vi "ERROR_DIALOGUE.vi"(0 "String":string) -> ()   [LabVIEW 2018]
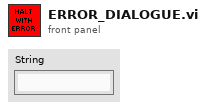
[diagram p1: front panel]
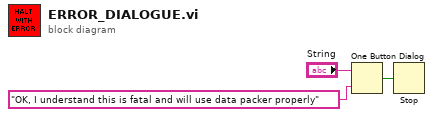
[diagram p0: block diagram]
diagram:
  n1 = One Button Dialog(message="String", button name ("OK")="OK, I understand this is fatal and will use data packer properly") -> (true=w1:bool)
  n2 = Stop(stop? (T)=w1) -> ()
